vi "Login.vi"(8 "error in (no error)":errorcluster, 10 "Authentication Inputs":T1, 11 "FormAuthentication in":refnum<class "FormAuthentication.lvclass">) -> (0 "error out":errorcluster, 2 "Authentication Outputs":T2, 3 "FormAuthentication out":refnum<class "FormAuthentication.lvclass">)   [LabVIEW 2020, in "HTTP Server.lvlib" / "FormAuthentication.lvclass"]
uses:
  FormAuthentication.lvclass
  lv-http-util/HTTP Utils/Request/Request.lvclass
  lv-http-util/HTTP Utils/FormField/FormField.lvclass
  HTTP Server.lvlib
  User/User.lvclass
  Session/Session.lvclass
  Authentication Outputs.ctl
  User Provider/User Provider.lvclass
  Password Encoder/Password Encoder.lvclass
  Authentication Inputs.ctl
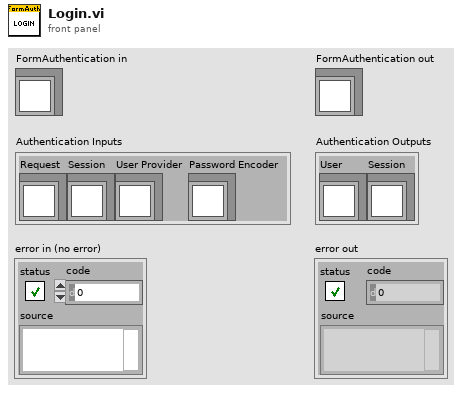
[diagram p1: front panel]
types:
  T1 = typedef "HTTP Server.lvlib/Authentication Inputs.ctl" = cluster{"Request":refnum<class "Request.lvclass">, "Session":refnum<class "Session.lvclass">, "User Provider":refnum<class "User Provider.lvclass">, "Password Encoder":refnum<class "Password Encoder.lvclass">}
  T2 = typedef "HTTP Server.lvlib/Authentication Outputs.ctl" = cluster{"User":refnum<class "User.lvclass">, "Session":refnum<class "Session.lvclass">}
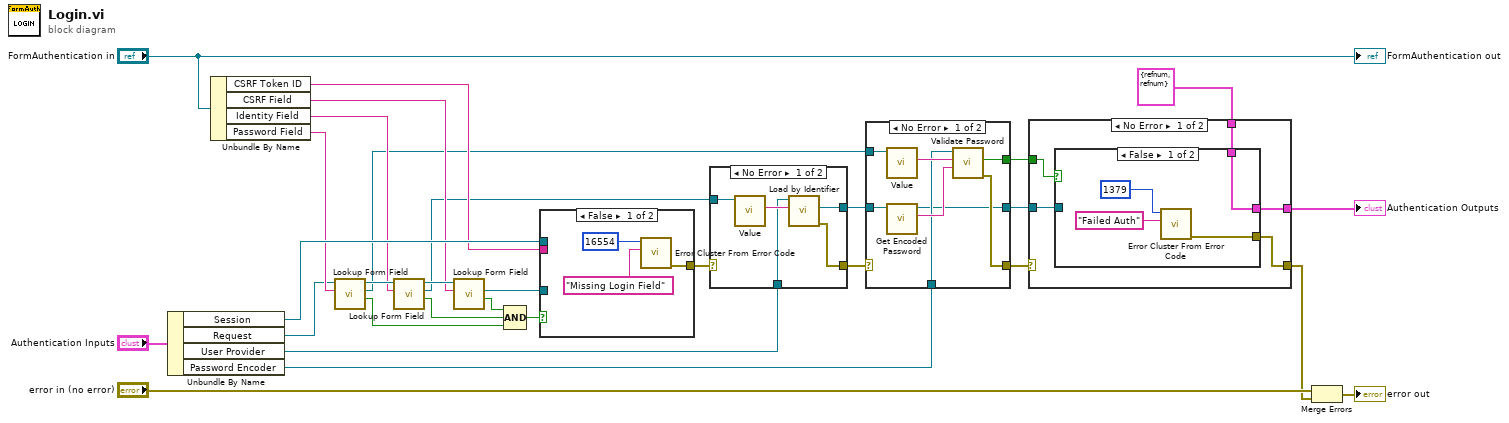
[diagram p0: block diagram]
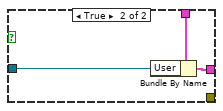
[diagram p2: hidden frame]
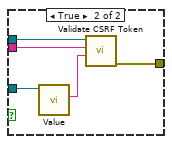
[diagram p6: hidden frame]
diagram:
  n1 = Unbundle By Name("Authentication Inputs") -> ("Session"=w21:refnum<class "Session.lvclass">, "Request"=w2:refnum<class "Request.lvclass">, "User Provider"=w14:refnum<class "User Provider.lvclass">, "Password Encoder"=w10:refnum<class "Password Encoder.lvclass">)
  n2 = Unbundle By Name("FormAuthentication in") -> ("CSRF Token ID"=w19:string, "CSRF Field"=w20:string, "Identity Field"=w18:string, "Password Field"=w17:string)
  n3 = call "Lookup Form Field.vi"("Name"=w17, "Request in"=w2) -> ("Exists"=w24:bool, "Field"=w12:refnum<class "FormField.lvclass">, "Request out"=w28:refnum<class "Request.lvclass">)  [unwired: 6 in, 1 out]
  n4 = call "Lookup Form Field.vi"("Name"=w18, "Request in"=w28) -> ("Exists"=w25:bool, "Field"=w15:refnum<class "FormField.lvclass">, "Request out"=w27:refnum<class "Request.lvclass">)  [unwired: 6 in, 1 out]
  n5 = call "Lookup Form Field.vi"("Name"=w20, "Request in"=w27) -> ("Exists"=w26:bool, "Field"=w22:refnum<class "FormField.lvclass">)  [unwired: 6 in, 2 out]
  n6 = Compound Arithmetic op=AND(w26, w25, w24) -> (w23:bool)
  n7 = case shown="False" w23 {
    tunnel: w22 -> [_ w38]
    tunnel: w21 -> [_ w37]
    tunnel: w19 -> [_ w36]
    tunnel: [w33 w34] -> w16
    frame False {
      n8 = call <vilib>:"Error Cluster From Error Code.vi"("error message (\"\")"="Missing Login Field" ("error message (\"\")"), "error code (0)"=16554) -> ("error out"=w33:errorcluster)  [unwired: 7 in]
    }
    frame True {
      n9 = call "Value.vi"("FormField in"=w38) -> ("Value"=w35:string)  [unwired: 8 in, 2 out]
      n10 = call "Validate CSRF Token.vi"("Token"=w35, "Token ID"=w36, "Session In"=w37) -> ("error out"=w34:errorcluster)  [unwired: 7 in, 1 out]
    }
  }
  n11 = case shown="No Error" w16 {
    selector: w16 -> [_ w44]
    tunnel: w15 -> [w43 _]
    tunnel: w14 -> [w41 _]
    tunnel: [w40 w44] -> w13
    tunnel: [w39 _] -> w11
    frame No Error {
      n12 = call "Value.vi"("FormField in"=w43) -> ("Value"=w42:string)  [unwired: 8 in, 2 out]
      n13 = call-dynamic "Load by Identifier.vi"("Identifier"=w42, "User Provider in"=w41) -> ("error out"=w40:errorcluster, "User"=w39:refnum<class "User.lvclass">)  [unwired: 7 in, 1 out]
    }
    frame Error {
    }
  }
  n14 = case shown="No Error" w13 {
    selector: w13 -> [_ w53]
    tunnel: w12 -> [w52 _]
    tunnel: w11 -> [w50 _]
    tunnel: w10 -> [w48 _]
    tunnel: [w47 w53] -> w9
    tunnel: [w46 _] -> w7
    tunnel: [w45 _] -> w8
    frame No Error {
      n15 = call "Value.vi"("FormField in"=w52) -> ("Value"=w51:string)  [unwired: 8 in, 2 out]
      n16 = call-dynamic "Get Encoded Password.vi"("User in"=w50) -> ("Encoded Password"=w49:string, "User out"=w45:refnum<class "User.lvclass">)  [unwired: 8 in, 1 out]
      n17 = call-dynamic "Validate Password.vi"("Encoded Password"=w49, "Plain Password"=w51, "Password Encoder in"=w48) -> ("error out"=w47:errorcluster, "Valid"=w46:bool)  [unwired: 6 in, 1 out]
    }
    frame Error {
    }
  }
  n18 = case shown="No Error" w9 {
    selector: w9 -> [_ w67]
    tunnel: w8 -> [w56 _]
    tunnel: w7 -> [w57 _]
    tunnel: [w54 w67] -> w3
    tunnel: T2 {"User"=refnum, "Session"=refnum} ("Authentication Outputs") -> [w58 w66]
    tunnel: [w55 w66] -> w5
    frame No Error {
      n19 = case shown="False" w57 {
        tunnel: w58 -> [w62 w65]
        tunnel: w56 -> [_ w64]
        tunnel: [w62 w63] -> w55
        tunnel: [w59 _] -> w54
        frame False {
          n20 = call <vilib>:"Error Cluster From Error Code.vi"("error message (\"\")"="Failed Auth" ("error message (\"\")"), "error code (0)"=1379) -> ("error out"=w59:errorcluster)  [unwired: 7 in]
        }
        frame True {
          n21 = Bundle By Name(cluster=w65, "User"=w64) -> (w63:T2)
        }
      }
    }
    frame Error {
    }
  }
  "Authentication Outputs" <- w5
  n22 = Merge Errors("error in (no error)", w3) -> (→"error out":errorcluster)
  "FormAuthentication out" <- "FormAuthentication in"
